vi "Check Existing Values SubVI.vi"(10 "Previous Value":string[](array[string]), 11 "String Array from Variable":string[](array[string])) -> (3 "String Array":string[](array[string]))   [LabVIEW 2014]
doc: "This subVI takes the previous string, checks the previous array and if there is any element that is the same in the previous array, it will not include it in the array of strings."
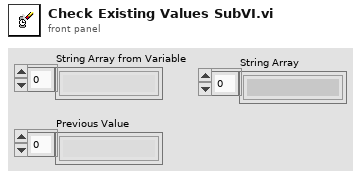
[diagram p1: front panel]
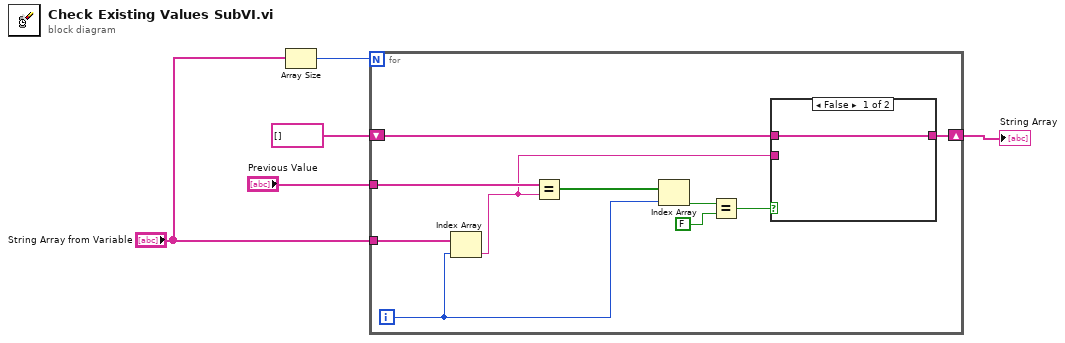
[diagram p0: block diagram]
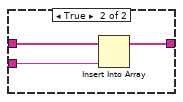
[diagram p2: hidden frame]
diagram:
  n1 = Array Size(array="String Array from Variable") -> (size(s)=w4:i32)
  n2 = for {
    N: w4 -> [_]
    tunnel: "String Array from Variable" -> [w15]
    tunnel: "Previous Value" -> [w14]
    shift-right: [w6] -> w1
    shift-left: string[] [] -> [w8]
    i -> [w12]
    n3 = Index Array(array=w15, index=w12) -> (element=w7:string)
    n4 = Equal?(x=w14, y=w7) -> (x = y?=w13:bool[])
    n5 = Index Array(array=w13, index=w12) -> (element=w11:bool)
    n6 = Equal?(x=w11, y=FALSE) -> (x = y?=w9:bool)
    n7 = case shown="False" w9 {
      tunnel: w8 -> [w16 w19]
      tunnel: w7 -> [_ w18]
      tunnel: [w16 w17] -> w6
      frame False {
      }
      frame True {
        n8 = Insert Into Array(array=w19, new element=w18) -> (w17:string[])  [unwired: 1 in]
      }
    }
  }
  "String Array" <- w1
